vi "Write KPRO Data cells to excel.vi"(0 "NI_report in":refnum<class "NI_report.lvclass">, 1 "milliseconds to wait":u32=100, 2 "all rows":string[][](array[string]), 3 "Row Offset In":i32=2, 5 "error in (no error)":errorcluster, 6 "Worksheet Names":string[](array[string])) -> (14 "NI_report out":refnum<class "NI_report.lvclass">, 16 "Row Offset Out":i32, 19 "error out":errorcluster)   [LabVIEW 2016]
uses:
  <vilib>/Utility/NIReport.llb/NI_report.lvclass
panel:
  out "number of rows":i32
  out "size(s)":i32[](array[numeric])
  in  "Current Sample Sheet":string="Processed Ik"
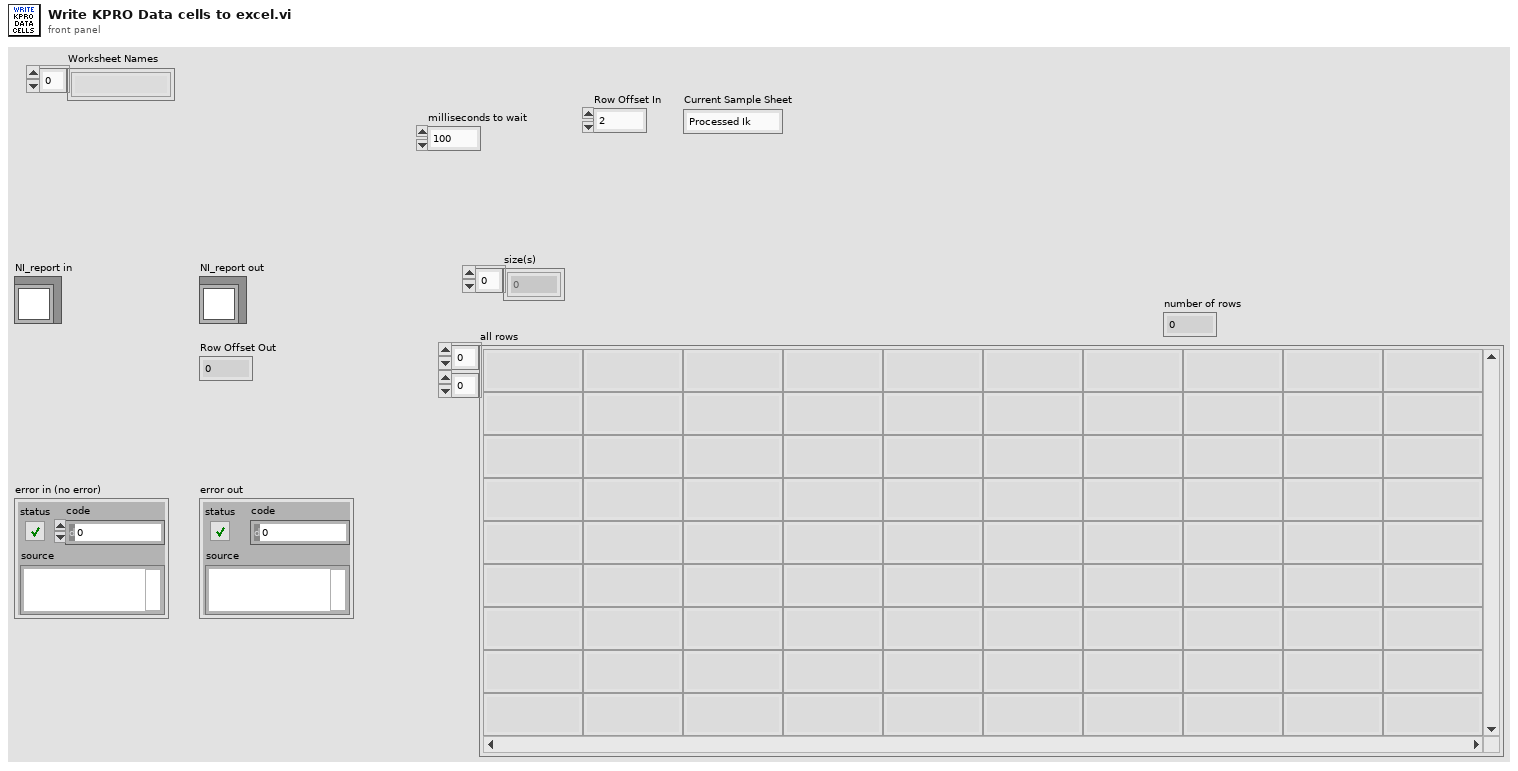
[diagram p1: front panel]
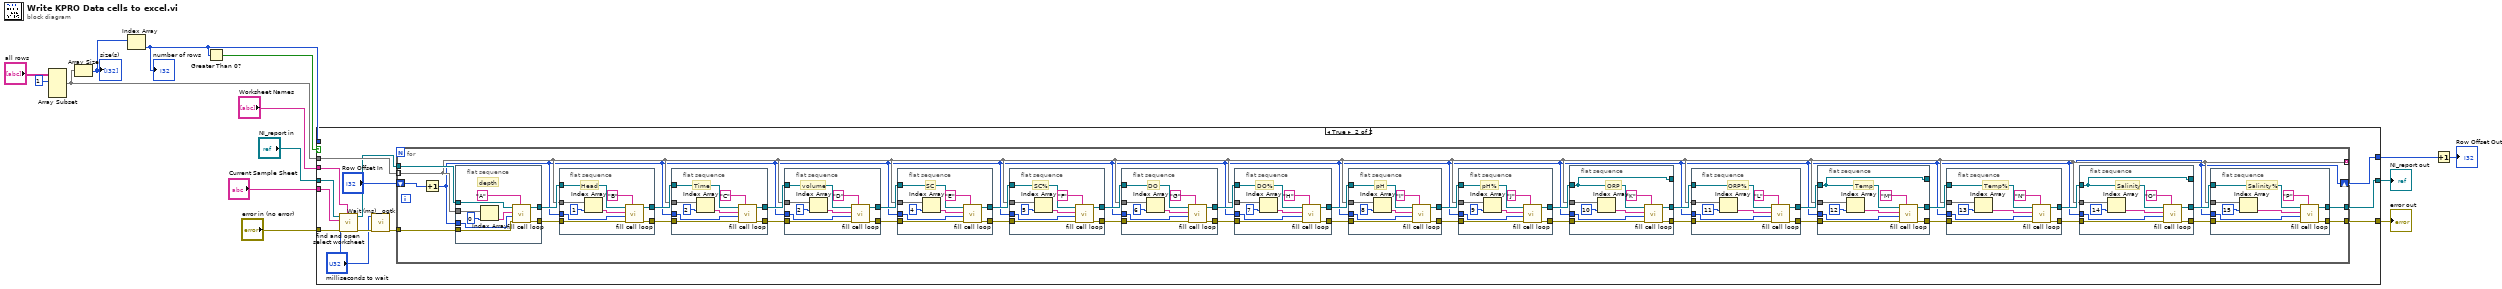
[diagram p0: block diagram]
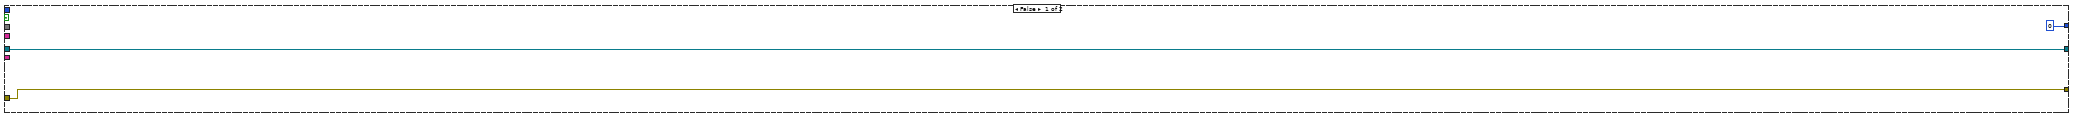
[diagram p2: hidden frame]
diagram:
  n1 = Array Subset(array="all rows", index (row)=1 ("index")) -> (w4:string[][])  [unwired: 3 in]
  n2 = Array Size(array=w4) -> (size(s)=w3:i32[])
  "size(s)" <- w3
  n3 = Index Array(array=w3) -> (element=w2:i32)  [unwired: 1 in]
  "number of rows" <- w2
  n4 = Greater Than 0?(x=w2) -> (x > 0?=w8:bool)
  n5 = case shown="True" w8 {
    tunnel: [w16 w30] -> w14
    tunnel: [w17 w29] -> w13
    tunnel: [0 ("Row Offset In") w28] -> w12
    tunnel: "NI_report in" -> [w17 w25]
    tunnel: "error in (no error)" -> [w16 w21]
    tunnel: "Worksheet Names" -> [_ w24]
    tunnel: w4 -> [_ w26]
    tunnel: w2 -> [_ _]
    tunnel: "Current Sample Sheet" -> [_ w20]
    frame False {
    }
    frame True {
      n6 = call "find and open select worksheet.vi"("Worksheet Names"=w24, "error in (no error)"=w21, "milliseconds to wait"="milliseconds to wait", "Worksheet Name in"=w20, "NI_report in"=w25) -> ("error out"=w22:errorcluster, "NI_report out"=w23:refnum<class "NI_report.lvclass">)  [unwired: 4 in, 1 out]
      n7 = call "Wait (ms)__ogtk.vi"("error in (no error)"=w22, "milliseconds to wait"="milliseconds to wait") -> ("error out"=w19:errorcluster)  [unwired: 8 in, 1 out]
      n8 = for {
        tunnel: w26 -> [w34] mode=indexing
        shift-right: [w33] -> w28
        shift-left: "Row Offset In" -> [w67]
        tunnel: w23 -> [w64]
        tunnel: w19 -> [w66]
        tunnel: [w32] -> w30
        tunnel: [w31] -> w29
        tunnel: [w34] -> _ mode=indexing
        n9 = Increment(x=w67) -> (x+1=w33:i32)
        n10 = flat-sequence {
          tunnel: w34 -> [w210]
          tunnel: w66 -> [w209]
          tunnel: [w208] -> w65
          tunnel: w33 -> [w207]
          tunnel: w64 -> [w205]
          tunnel: [w204] -> w63
          frame #0 {
            # "depth"
            n11 = Index Array(array=w210, index=0) -> (element=w206:string)
            n12 = call "fill cell loop.vi"("Column Letter"="A" ("Depth Column Letter"), "error in (no error)"=w209, "Row"=w207, "String"=w206, "NI_report in"=w205) -> ("error out"=w208:errorcluster, "NI_report out"=w204:refnum<class "NI_report.lvclass">)  [unwired: 5 in]
          }
        }
        n13 = flat-sequence {
          tunnel: [w202] -> w61
          tunnel: [w201] -> w62
          tunnel: w34 -> [w197]
          tunnel: w65 -> [w196]
          tunnel: w33 -> [w195]
          tunnel: w63 -> [w194]
          frame #0 {
            # "Head"
            n14 = Index Array(array=w197, index=1) -> (element=w198:string)
            n15 = call "fill cell loop.vi"("Column Letter"="B" ("Head Column Letter"), "error in (no error)"=w196, "Row"=w195, "String"=w198, "NI_report in"=w194) -> ("error out"=w202:errorcluster, "NI_report out"=w201:refnum<class "NI_report.lvclass">)  [unwired: 5 in]
          }
        }
        n16 = flat-sequence {
          tunnel: [w193] -> w59
          tunnel: [w192] -> w60
          tunnel: w34 -> [w188]
          tunnel: w61 -> [w187]
          tunnel: w33 -> [w186]
          tunnel: w62 -> [w185]
          frame #0 {
            # "Time"
            n17 = Index Array(array=w188, index=2) -> (element=w189:string)
            n18 = call "fill cell loop.vi"("Column Letter"="C" ("Head Column Letter"), "error in (no error)"=w187, "Row"=w186, "String"=w189, "NI_report in"=w185) -> ("error out"=w193:errorcluster, "NI_report out"=w192:refnum<class "NI_report.lvclass">)  [unwired: 5 in]
          }
        }
        n19 = flat-sequence {
          tunnel: [w184] -> w57
          tunnel: [w183] -> w58
          tunnel: w34 -> [w179]
          tunnel: w59 -> [w178]
          tunnel: w33 -> [w177]
          tunnel: w60 -> [w176]
          frame #0 {
            # "volume"
            n20 = Index Array(array=w179, index=2) -> (element=w180:string)
            n21 = call "fill cell loop.vi"("Column Letter"="D" ("Head Column Letter"), "error in (no error)"=w178, "Row"=w177, "String"=w180, "NI_report in"=w176) -> ("error out"=w184:errorcluster, "NI_report out"=w183:refnum<class "NI_report.lvclass">)  [unwired: 5 in]
          }
        }
        n22 = flat-sequence {
          tunnel: [w175] -> w55
          tunnel: [w174] -> w56
          tunnel: w34 -> [w170]
          tunnel: w57 -> [w169]
          tunnel: w33 -> [w168]
          tunnel: w58 -> [w167]
          frame #0 {
            # "SC"
            n23 = Index Array(array=w170, index=4) -> (element=w171:string)
            n24 = call "fill cell loop.vi"("Column Letter"="E" ("Head Column Letter"), "error in (no error)"=w169, "Row"=w168, "String"=w171, "NI_report in"=w167) -> ("error out"=w175:errorcluster, "NI_report out"=w174:refnum<class "NI_report.lvclass">)  [unwired: 5 in]
          }
        }
        n25 = flat-sequence {
          tunnel: [w166] -> w51
          tunnel: [w165] -> w52
          tunnel: w34 -> [w161]
          tunnel: w55 -> [w160]
          tunnel: w33 -> [w159]
          tunnel: w56 -> [w158]
          frame #0 {
            # "SC%"
            n26 = Index Array(array=w161, index=5) -> (element=w162:string)
            n27 = call "fill cell loop.vi"("Column Letter"="F" ("Head Column Letter"), "error in (no error)"=w160, "Row"=w159, "String"=w162, "NI_report in"=w158) -> ("error out"=w166:errorcluster, "NI_report out"=w165:refnum<class "NI_report.lvclass">)  [unwired: 5 in]
          }
        }
        n28 = flat-sequence {
          tunnel: [w157] -> w54
          tunnel: [w156] -> w53
          tunnel: w34 -> [w152]
          tunnel: w51 -> [w151]
          tunnel: w33 -> [w150]
          tunnel: w52 -> [w149]
          frame #0 {
            # "DO"
            n29 = Index Array(array=w152, index=6) -> (element=w153:string)
            n30 = call "fill cell loop.vi"("Column Letter"="G" ("Head Column Letter"), "error in (no error)"=w151, "Row"=w150, "String"=w153, "NI_report in"=w149) -> ("error out"=w157:errorcluster, "NI_report out"=w156:refnum<class "NI_report.lvclass">)  [unwired: 5 in]
          }
        }
        n31 = flat-sequence {
          tunnel: [w148] -> w47
          tunnel: [w147] -> w48
          tunnel: w34 -> [w143]
          tunnel: w54 -> [w142]
          tunnel: w33 -> [w141]
          tunnel: w53 -> [w140]
          frame #0 {
            # "DO%"
            n32 = Index Array(array=w143, index=7) -> (element=w144:string)
            n33 = call "fill cell loop.vi"("Column Letter"="H" ("Head Column Letter"), "error in (no error)"=w142, "Row"=w141, "String"=w144, "NI_report in"=w140) -> ("error out"=w148:errorcluster, "NI_report out"=w147:refnum<class "NI_report.lvclass">)  [unwired: 5 in]
          }
        }
        n34 = flat-sequence {
          tunnel: [w139] -> w49
          tunnel: [w138] -> w50
          tunnel: w34 -> [w134]
          tunnel: w47 -> [w133]
          tunnel: w33 -> [w132]
          tunnel: w48 -> [w131]
          frame #0 {
            # "pH"
            n35 = Index Array(array=w134, index=8) -> (element=w135:string)
            n36 = call "fill cell loop.vi"("Column Letter"="I" ("Head Column Letter"), "error in (no error)"=w133, "Row"=w132, "String"=w135, "NI_report in"=w131) -> ("error out"=w139:errorcluster, "NI_report out"=w138:refnum<class "NI_report.lvclass">)  [unwired: 5 in]
          }
        }
        n37 = flat-sequence {
          tunnel: [w130] -> w44
          tunnel: [w129] -> w43
          tunnel: w34 -> [w125]
          tunnel: w49 -> [w124]
          tunnel: w33 -> [w123]
          tunnel: w50 -> [w122]
          frame #0 {
            # "pH%"
            n38 = Index Array(array=w125, index=9) -> (element=w126:string)
            n39 = call "fill cell loop.vi"("Column Letter"="J" ("Head Column Letter"), "error in (no error)"=w124, "Row"=w123, "String"=w126, "NI_report in"=w122) -> ("error out"=w130:errorcluster, "NI_report out"=w129:refnum<class "NI_report.lvclass">)  [unwired: 5 in]
          }
        }
        n40 = flat-sequence {
          tunnel: [w121] -> w46
          tunnel: [w120] -> w45
          tunnel: w34 -> [w116]
          tunnel: w44 -> [w115]
          tunnel: w33 -> [w114]
          tunnel: [w113] -> _
          tunnel: w43 -> [w113]
          frame #0 {
            # "ORP"
            n41 = Index Array(array=w116, index=10) -> (element=w117:string)
            n42 = call "fill cell loop.vi"("Column Letter"="K" ("Head Column Letter"), "error in (no error)"=w115, "Row"=w114, "String"=w117, "NI_report in"=w113) -> ("error out"=w121:errorcluster, "NI_report out"=w120:refnum<class "NI_report.lvclass">)  [unwired: 5 in]
          }
        }
        n43 = flat-sequence {
          tunnel: [w112] -> w40
          tunnel: [w111] -> w39
          tunnel: w34 -> [w107]
          tunnel: w46 -> [w106]
          tunnel: w33 -> [w105]
          tunnel: w45 -> [w104]
          frame #0 {
            # "ORP%"
            n44 = Index Array(array=w107, index=11) -> (element=w108:string)
            n45 = call "fill cell loop.vi"("Column Letter"="L" ("Head Column Letter"), "error in (no error)"=w106, "Row"=w105, "String"=w108, "NI_report in"=w104) -> ("error out"=w112:errorcluster, "NI_report out"=w111:refnum<class "NI_report.lvclass">)  [unwired: 5 in]
          }
        }
        n46 = flat-sequence {
          tunnel: [w85] -> w36
          tunnel: [w84] -> w35
          tunnel: w34 -> [w80]
          tunnel: w40 -> [w79]
          tunnel: w33 -> [w78]
          tunnel: w39 -> [w77]
          tunnel: [w77] -> _
          frame #0 {
            # "Temp"
            n47 = Index Array(array=w80, index=12) -> (element=w81:string)
            n48 = call "fill cell loop.vi"("Column Letter"="M" ("Head Column Letter"), "error in (no error)"=w79, "Row"=w78, "String"=w81, "NI_report in"=w77) -> ("error out"=w85:errorcluster, "NI_report out"=w84:refnum<class "NI_report.lvclass">)  [unwired: 5 in]
          }
        }
        n49 = flat-sequence {
          tunnel: [w76] -> w37
          tunnel: [w75] -> w38
          tunnel: w34 -> [w71]
          tunnel: w33 -> [w70]
          tunnel: w36 -> [w69]
          tunnel: w35 -> [w68]
          frame #0 {
            # "Temp%"
            n50 = Index Array(array=w71, index=13) -> (element=w72:string)
            n51 = call "fill cell loop.vi"("Column Letter"="N" ("Head Column Letter"), "error in (no error)"=w69, "Row"=w70, "String"=w72, "NI_report in"=w68) -> ("error out"=w76:errorcluster, "NI_report out"=w75:refnum<class "NI_report.lvclass">)  [unwired: 5 in]
          }
        }
        n52 = flat-sequence {
          tunnel: [w103] -> w41
          tunnel: [w102] -> w42
          tunnel: w34 -> [w98]
          tunnel: w37 -> [w97]
          tunnel: w33 -> [w96]
          tunnel: w38 -> [w95]
          tunnel: [w95] -> _
          frame #0 {
            # "Salinity"
            n53 = Index Array(array=w98, index=14) -> (element=w99:string)
            n54 = call "fill cell loop.vi"("Column Letter"="O" ("Head Column Letter"), "error in (no error)"=w97, "Row"=w96, "String"=w99, "NI_report in"=w95) -> ("error out"=w103:errorcluster, "NI_report out"=w102:refnum<class "NI_report.lvclass">)  [unwired: 5 in]
          }
        }
        n55 = flat-sequence {
          tunnel: [w94] -> w32
          tunnel: [w93] -> w31
          tunnel: w34 -> [w89]
          tunnel: w41 -> [w88]
          tunnel: w33 -> [w87]
          tunnel: w42 -> [w86]
          frame #0 {
            # "Salinity%"
            n56 = Index Array(array=w89, index=15) -> (element=w90:string)
            n57 = call "fill cell loop.vi"("Column Letter"="P" ("Head Column Letter"), "error in (no error)"=w88, "Row"=w87, "String"=w90, "NI_report in"=w86) -> ("error out"=w94:errorcluster, "NI_report out"=w93:refnum<class "NI_report.lvclass">)  [unwired: 5 in]
          }
        }
      }
    }
  }
  "error out" <- w14
  "NI_report out" <- w13
  n58 = Increment(x=w12) -> (x+1=→"Row Offset Out":i32)
